vi "Win Host - dialog_1bt.vi"(7 "Language":T1, 8 "error in (no error)":errorcluster, 11 "Message":string caption="AI analysis is not ready yet.") -> (0 "error out":errorcluster, 3 "Exit?":bool)   [LabVIEW 2024]
uses:
  Buttons/Cancel.ctl
  Buttons/OK.ctl
  Controls/Language.ctl
  <vilib>/addons/Tools/Unicode/UI Unicode Tools.lvlib
panel:
  in  "OK Button":T2
  in  "Cancel Button":T3
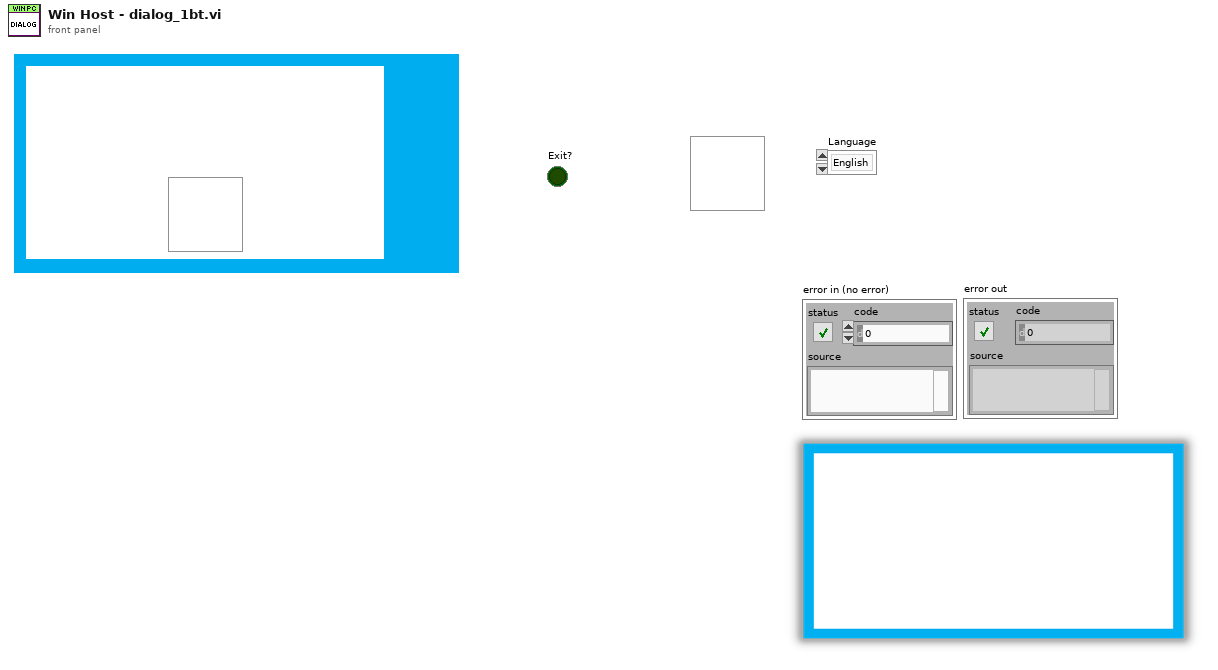
[diagram p1: front panel]
types:
  T1 = typedef "Language.ctl" = enum16{"English", "Chinese", "German"}
  T2 = typedef "OK.ctl" = bool
  T3 = typedef "Cancel.ctl" = bool
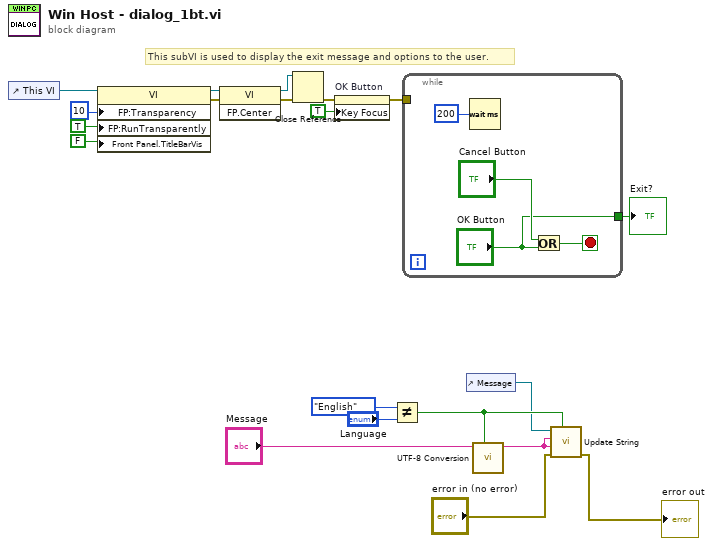
[diagram p0: block diagram]
diagram:
  # "This subVI is used to display the exit message and options to the user."
  n1 = control-ref of="This VI"() -> (w18:refnum<vi>)
  n2 = property class="VI"(reference=w18, "FP:Transparency"=u8 10 ("Front Panel Window:Transparency"), "FP:RunTransparently"=TRUE ("Front Panel Window:Title Bar Visible"), "Front Panel.TitleBarVis"=FALSE ("Front Panel Window:Title Bar Visible")) -> (reference out=w16:refnum<vi>, error out=w15:errorcluster)  [unwired: 1 in]
  n3 = invoke class="VI" method="FP.Center"(reference=w16, error in=w15) -> (reference out=w20:refnum<vi>, error out=w19:errorcluster)  [unwired: 1 in, 1 out]
  n4 = Close Reference(reference=w20, error in (no error)=w19) -> (error out=w10:errorcluster)
  n5 = property on="OK Button" class="Bool"(error in=w10, "Key Focus"=TRUE) -> (error out=w9:errorcluster)  [unwired: 1 in, 1 out]
  n6 = Not Equal?(x=Language."English" ("UI Information.Language"), y="Language") -> (x != y?=w5:bool)
  n7 = while {
    tunnel: ["OK Button"] -> w12
    tunnel: w9 -> [_]
    stop <- w23 stop-if-true
    n8 = Wait (ms)(milliseconds to wait=u32 200) -> ()  [unwired: 1 out]
    n9 = Or(x="Cancel Button", y="OK Button") -> (x .or. y?=w23:T3)
  }
  "Exit?" <- w12
  n10 = control-ref of="Message"() -> (w4:refnum<vi>)
  n11 = call "UTF-8 Conversion.vi"("Unicode?"=w5, "Config String"="Message") -> ("Unicode/ANSI string"=w8:string)  [unwired: 8 in, 1 out]
  n12 = call <vilib>:"Update String.vi"("Interpret as Unicode (T)"=w5, "error in (no error)"="error in (no error)", "Caption"=w8, "String Value"=w8, "String Control Reference"=w4) -> ("error out"=→"error out":errorcluster)  [unwired: 3 in, 1 out]
